vi "Generate_WayPoints_Hopping WITH VariableV2Patterning.vi"(11 "Input Cluster":T2={"Scan Rate (um/s)"=15.0, "X Start"=15.0, "X End"=15.0, "Y Start"=15.0, "Y End"=15.0, " Z Start"=15.0, "HoppingDistance"=1.0, "Voltage1"=15.0, "Z End"=15.0, "Approach Rate Hopping (um/s)"=15.0, "Retrack Rate (um/s)"=15.0, "Voltage2"=15.0, "Approach Rate (um/s)"=15.0, "Hold Time START / s"=15.0, "Hold Time Delta / s"=15.0, "Voltage1 During Retract"=0.0, "Pause on First Approach?"=FALSE, "Voltage2 During Retract"=0.0, "Voltage1 During Hold Time"=0.0, "Voltage2 During Hold Time"=0.0, "Update position loop wait time (us)"=0}) -> (1 "output cluster":T1)   [LabVIEW 2023]
uses:
  TypeDefs/WayPointCluster.ctl
  User_Vi/Settings.vi
panel:
  in  "WayPointCluster":T1
  out "Y  P":dbl
  out "X  P":dbl
  out "HoppingDistanceX":dbl
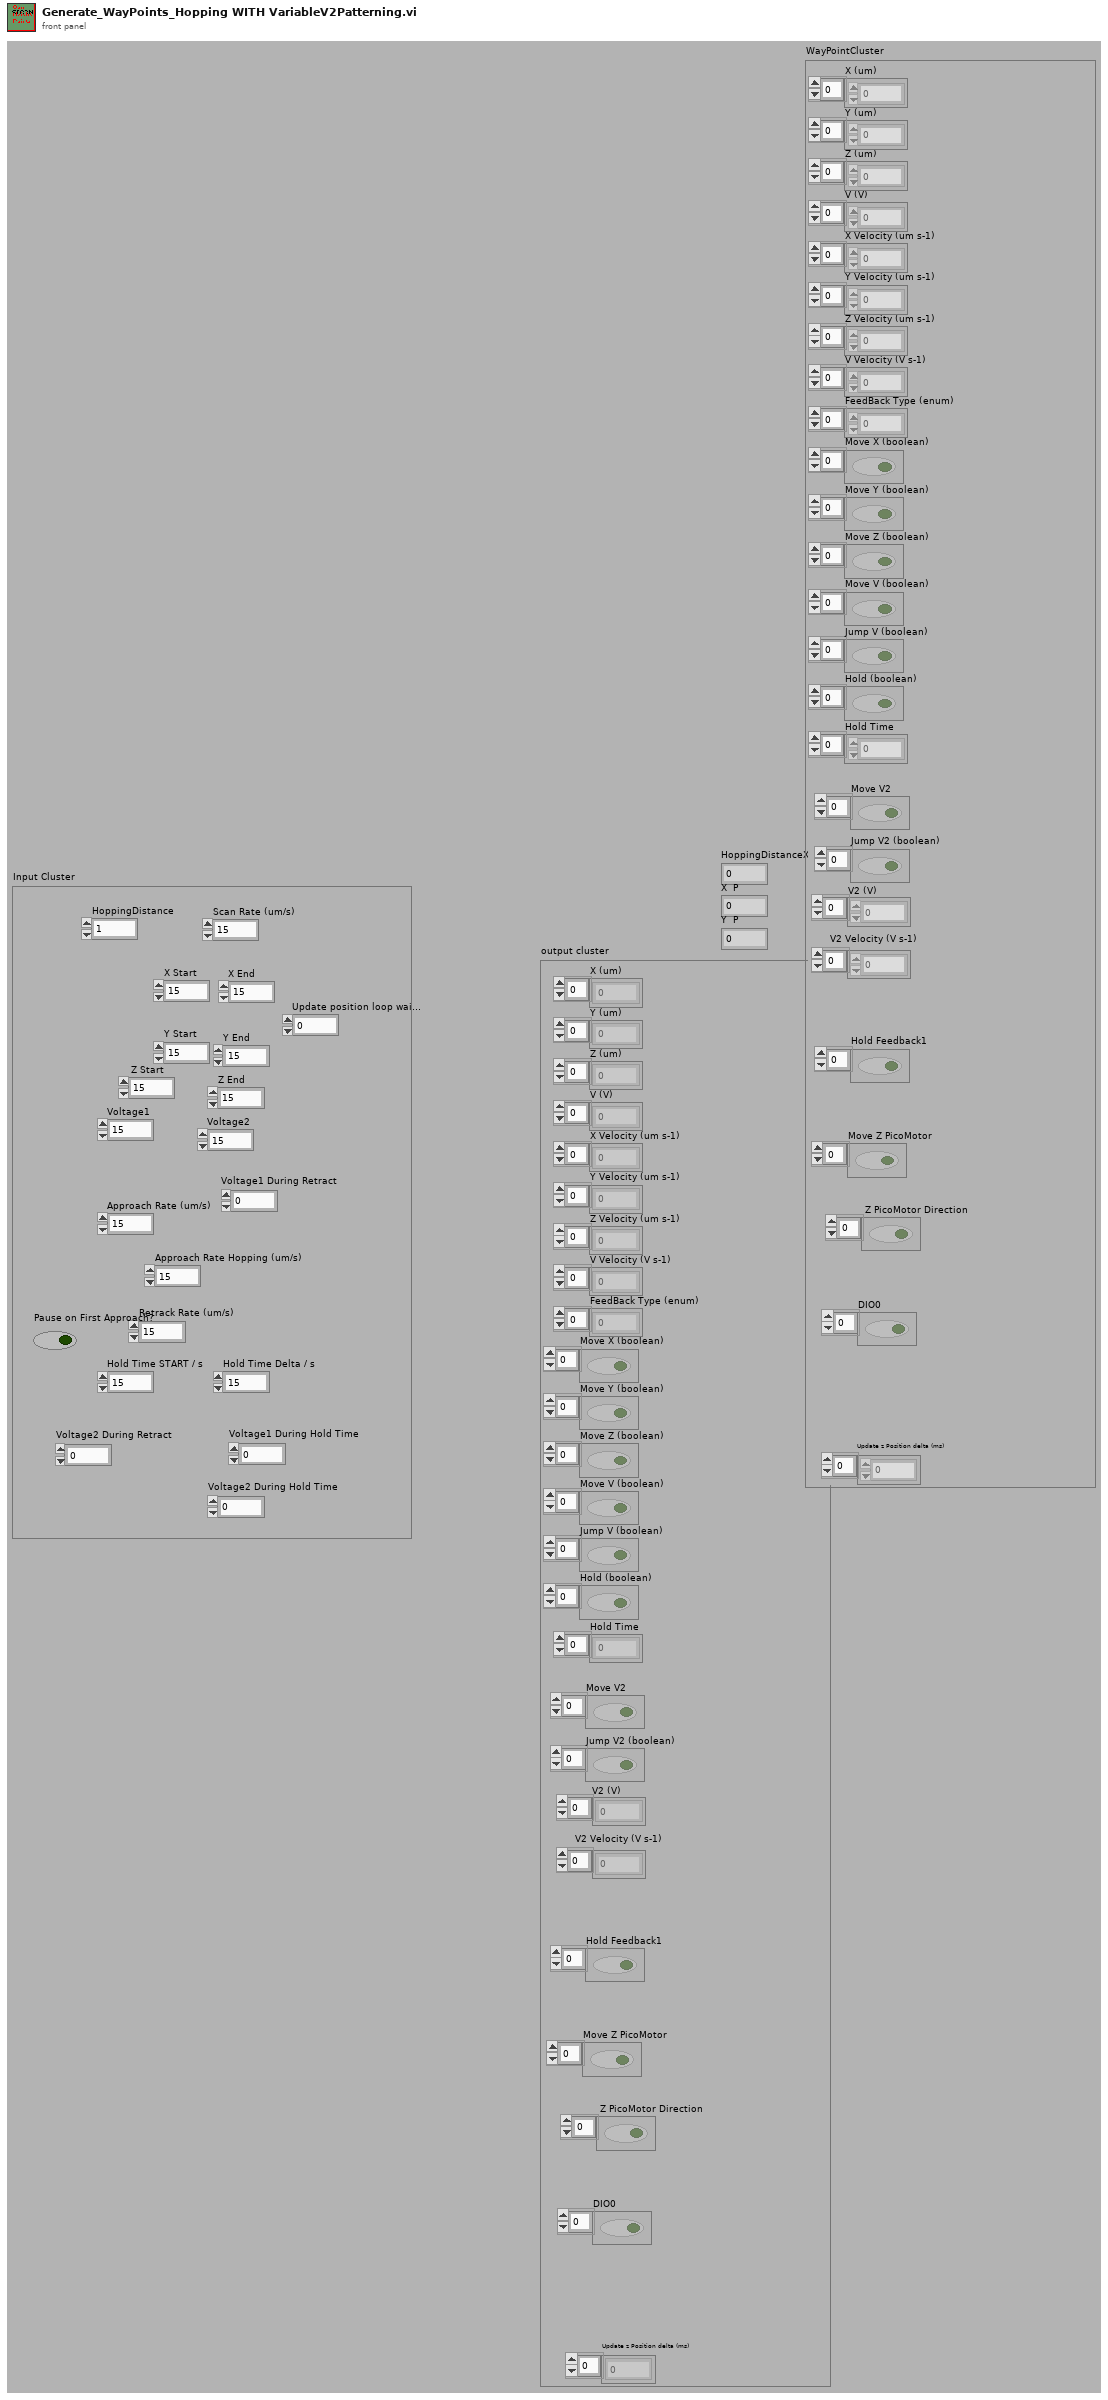
[diagram p1: front panel]
types:
  T1 = typedef "WayPointCluster.ctl" = cluster{"X (um)":dbl[], "Y (um)":dbl[], "Z (um)":dbl[], "V (V)":dbl[], "X Velocity (um s-1)":dbl[], "Y Velocity (um s-1)":dbl[], "Z Velocity (um s-1)":dbl[], "V Velocity (V s-1)":dbl[], "FeedBack Type (enum)":u16[], "Move X (boolean)":bool[], "Move Y (boolean)":bool[], "Move Z (boolean)":bool[], "Move V (boolean)":bool[], "Jump V (boolean)":bool[], "Hold (boolean)":bool[], "Hold Time":u32[], "V2 (V)":dbl[], "Move V2":bool[], "V2 Velocity (V s-1)":dbl[], "Jump V2 (boolean)":bool[], "Update z Position delta (ms)":i16[], "Hold Feedback1":bool[], "Move Z PicoMotor":bool[], " Z PicoMotor Direction":bool[], "DIO0":bool[]}
  T2 = cluster{"Scan Rate (um/s)":dbl, "X Start":dbl, "X End":dbl, "Y Start":dbl, "Y End":dbl, " Z Start":dbl, "HoppingDistance":dbl, "Voltage1":dbl, "Z End":dbl, "Approach Rate Hopping (um/s)":dbl, "Retrack Rate (um/s)":dbl, "Voltage2":dbl, "Approach Rate (um/s)":dbl, "Hold Time START / s":dbl, "Hold Time Delta / s":dbl, "Voltage1 During Retract":dbl, "Pause on First Approach?":bool, "Voltage2 During Retract":dbl, "Voltage1 During Hold Time":dbl, "Voltage2 During Hold Time":dbl, "Update position loop wait time (us)":u32}
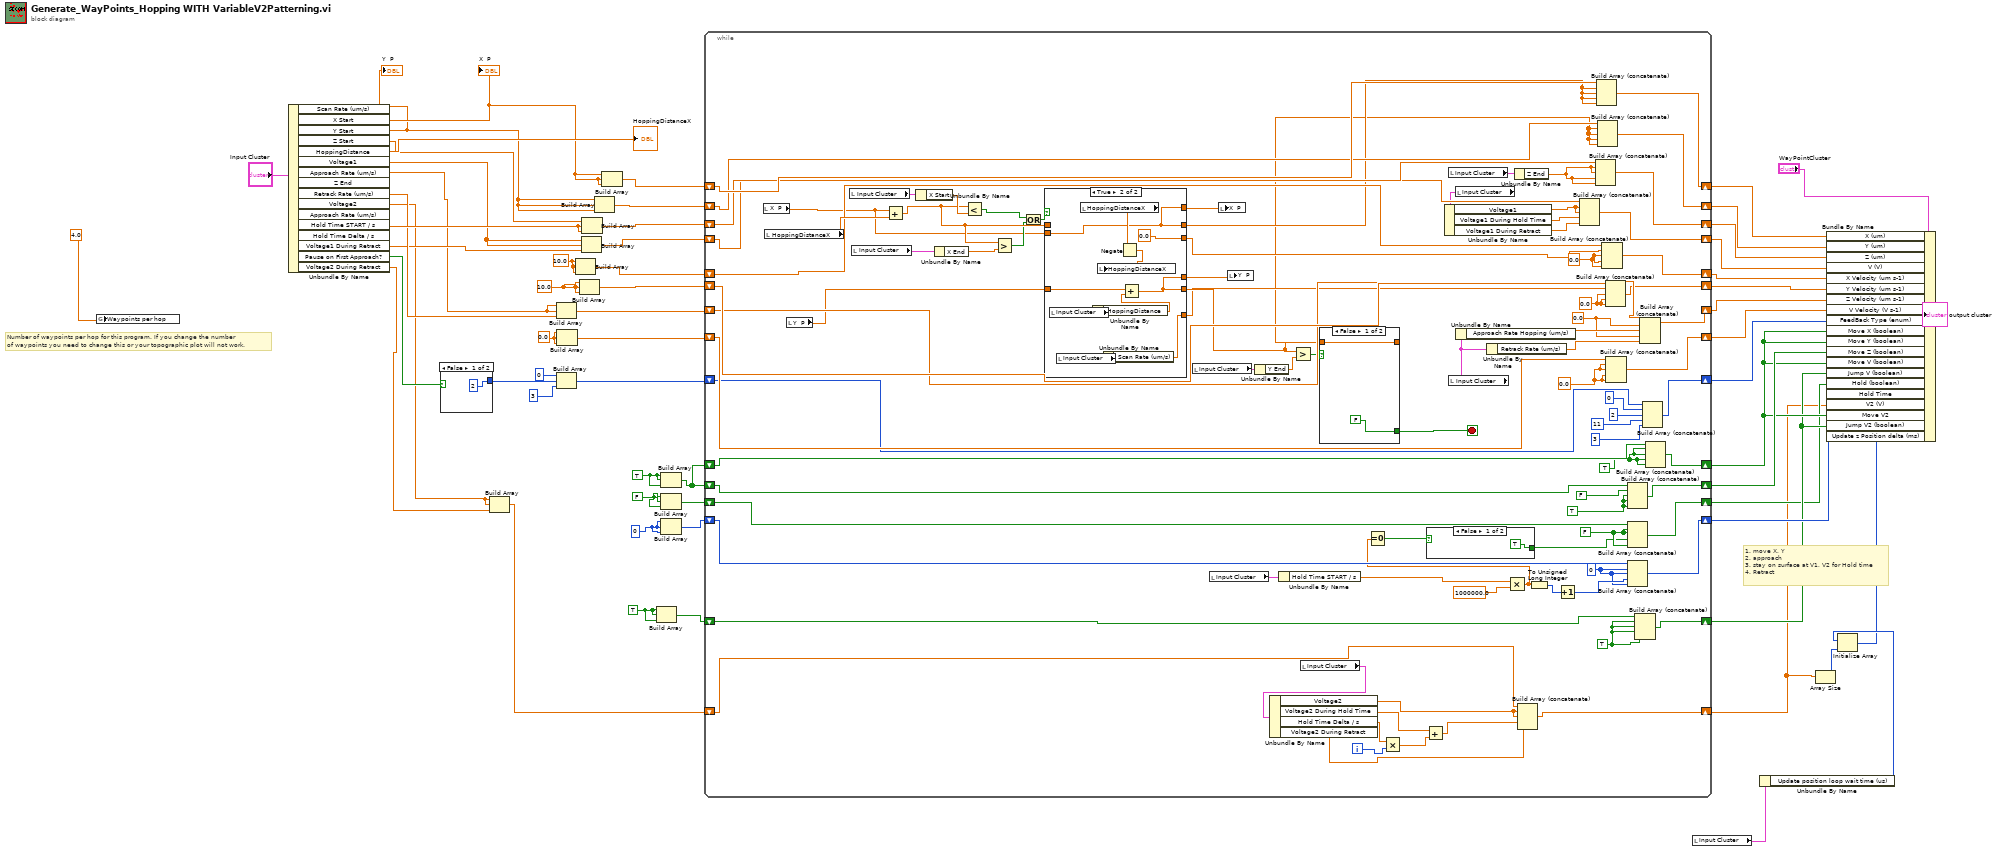
[diagram p0: block diagram]
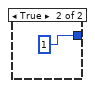
[diagram p2: hidden frame]
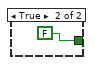
[diagram p3: hidden frame]
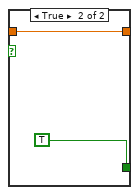
[diagram p4: hidden frame]
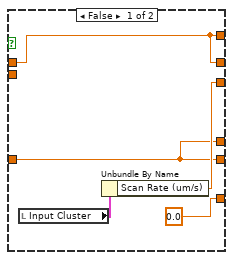
[diagram p5: hidden frame]
diagram:
  w22 = TRUE
  w23 = u32 0 ("element")
  w24 = FALSE
  w25 = TRUE
  w18 = 10.0 ("element")
  w19 = 10.0 ("element")
  w21 = 0.0 ("element")
  # "1. move X, Y\n2. approach\n3. stay on surface at V1, V2 for Hold time \n4. Retract"
  # "Number of waypoints per hop for this program. If you change the number\nof waypoints you need to change this or your topographic plot will not work."
  n1 = global write "Settings.vi" "Waypoints per hop"(4.0) -> ()
  n2 = Unbundle By Name("Input Cluster") -> ("X Start"=w39:dbl, "Y Start"=w38:dbl, "Z Start"=w40:dbl, "HoppingDistance"=→"HoppingDistanceX":dbl, "Voltage1"=w36:dbl, "Approach Rate (um/s)"=w20:dbl, "Z End"=w37:dbl, "Retrack Rate (um/s)"=w35:dbl, "Voltage2"=w12:dbl, "Voltage1 During Retract"=w27:dbl, "Pause on First Approach?"=w15:bool, "Voltage2 During Retract"=w11:dbl)  [unwired: 4 out]
  "X  P" <- w39
  "Y  P" <- w38
  n3 = case shown="False" w15 {
    tunnel: [u16 2 ("element") u16 1 ("element")] -> w14
    frame False {
    }
    frame True {
    }
  }
  n4 = Build Array(w12, w12, w11) -> (w8:dbl[])
  n5 = Build Array(w20, w20, w35) -> (w47:dbl[])
  n6 = Build Array(u16 0 ("element"), w14, u16 3 ("element")) -> (w43:u16[])
  n7 = Build Array(w21, w21, w21) -> (w45:dbl[])
  n8 = Build Array(w18, w18, w18) -> (w50:dbl[])
  n9 = Build Array(w19, w19, w19) -> (w49:dbl[])
  n10 = Build Array(w36, w36, w27) -> (w52:dbl[])
  n11 = Build Array(w40, w37, w37) -> (w54:dbl[])
  n12 = Build Array(w38, w38, w38) -> (w56:dbl[])
  n13 = Build Array(w39, w39, w39) -> (w58:dbl[])
  n14 = Build Array(w22, w22, w22) -> (w29:bool[])
  n15 = Build Array(w25, w25, w25) -> (w28:bool[])
  n16 = Build Array(w24, w24, w24) -> (w32:bool[])
  n17 = Build Array(w23, w23, w23) -> (w31:u32[])
  n18 = while {
    shift-right: [w148] -> w57
    shift-left: w58 -> [w149]
    shift-right: [w140] -> w55
    shift-left: w56 -> [w130]
    shift-right: [w139] -> w53
    shift-left: w54 -> [w147]
    shift-right: [w138] -> w51
    shift-left: w52 -> [w146]
    shift-right: [w137] -> w33
    shift-left: w50 -> [w145]
    shift-right: [w136] -> w48
    shift-left: w49 -> [w144]
    shift-right: [w135] -> w46
    shift-left: w47 -> [w143]
    shift-right: [w134] -> w44
    shift-left: w45 -> [w142]
    shift-right: [w133] -> w42
    shift-left: w43 -> [w141]
    shift-right: [w104] -> w13
    shift-left: w28 -> [w103]
    shift-right: [w105] -> w6
    shift-left: w32 -> [w109]
    shift-right: [w106] -> w30
    shift-left: w31 -> [w108]
    shift-right: [w101] -> w9
    shift-left: w29 -> [w102]
    shift-right: [w99] -> w10
    shift-left: w28 -> [w100]
    shift-right: [w84] -> w5
    shift-left: w8 -> [w85]
    i -> [w66]
    stop <- w120 stop-if-true
    w73 = TRUE
    w71 = TRUE
    w92 = u32 0 ("element")
    w94 = FALSE
    w69 = TRUE
    w77 = 0.0 ("element")
    w78 = 0.0 ("element")
    w75 = 0.0 ("element")
    w76 = 0.0 ("element")
    n19 = local read "X  P"() -> (w118:dbl)
    n20 = local read "HoppingDistanceX"() -> (w150:dbl)
    n21 = local read "Y  P"() -> (w117:dbl)
    n22 = local read "Input Cluster"() -> (w152:T2)
    n23 = local read "Input Cluster"() -> (w151:T2)
    n24 = Add(x=w118, y=w150) -> (x+y=w126:dbl)
    n25 = Unbundle By Name(w152) -> ("X Start"=w129:dbl)
    n26 = Unbundle By Name(w151) -> ("X End"=w127:dbl)
    n27 = Less?(x=w126, y=w129) -> (x < y?=w128:bool)
    n28 = Greater?(x=w126, y=w127) -> (0:w125:bool)
    n29 = Or(x=w128, y=w125) -> (x .or. y?=w124:bool)
    n30 = case shown="True" w124 {
      tunnel: w126 -> [w159 _]
      tunnel: [w159 w165] -> w82
      tunnel: w118 -> [_ w165]
      tunnel: w117 -> [w160 w166]
      tunnel: [w160 w164] -> w116
      tunnel: [w162 0.0] -> w111
      tunnel: [0.0 w167] -> w110
      tunnel: [w160 w164] -> w115
      tunnel: [w159 w165] -> w114
      frame False {
        n31 = local read "Input Cluster"() -> (w163:T2)
        n32 = Unbundle By Name(w163) -> ("Scan Rate (um/s)"=w162:dbl)
      }
      frame True {
        n33 = local read "Input Cluster"() -> (w171:T2)
        n34 = local read "Input Cluster"() -> (w169:T2)
        n35 = local read "HoppingDistanceX"() -> (w173:dbl)
        n36 = Unbundle By Name(w171) -> ("HoppingDistance"=w170:dbl)
        n37 = Unbundle By Name(w169) -> ("Scan Rate (um/s)"=w167:dbl)
        n38 = Negate(x=w173) -> (-x=w172:dbl)
        n39 = local write "HoppingDistanceX"(w172) -> ()
        n40 = Add(x=w166, y=w170) -> (x+y=w164:dbl)
      }
    }
    n41 = local read "Input Cluster"() -> (w123:T2)
    n42 = local read "Input Cluster"() -> (w107:T2)
    n43 = local write "X  P"(w114) -> ()
    n44 = local write "Y  P"(w115) -> ()
    n45 = Unbundle By Name(w123) -> ("Y End"=w122:dbl)
    n46 = Unbundle By Name(w107) -> ("Hold Time START / s"=w67:dbl)
    n47 = Greater?(x=w116, y=w122) -> (0:w121:bool)
    n48 = local read "Input Cluster"() -> (w86:T2)
    n49 = Unbundle By Name(w86) -> ("Voltage2"=w83:dbl, "Voltage2 During Hold Time"=w63:dbl, "Hold Time Delta / s"=w65:dbl, "Voltage2 During Retract"=w68:dbl)
    n50 = case shown="False" w121 {
      tunnel: w116 -> [w156 w158]
      tunnel: [w156 w158] -> w81
      tunnel: [FALSE TRUE] -> w120
      frame False {
      }
      frame True {
      }
    }
    n51 = Multiply(x=w65, y=w66) -> (x*y=w64:dbl)
    n52 = Add(x=w63, y=w64) -> (x+y=w62:dbl)
    n53 = local read "Input Cluster"() -> (w132:T2)
    n54 = local read "Input Cluster"() -> (w119:T2)
    n55 = local read "Input Cluster"() -> (w131:T2)
    n56 = Unbundle By Name(w131) -> ("Voltage1"=w88:dbl, "Voltage1 During Hold Time"=w87:dbl, "Voltage1 During Retract"=w79:dbl)
    n57 = Unbundle By Name(w119) -> ("Approach Rate Hopping (um/s)"=w112:dbl)
    n58 = Unbundle By Name(w119) -> ("Retrack Rate (um/s)"=w96:dbl)
    n59 = Multiply(x=w67, y=1000000.0) -> (x*y=w89:dbl)
    n60 = Equal To 0?(x=w89) -> (x = 0?=w90:bool)
    n61 = case shown="False" w90 {
      tunnel: [TRUE FALSE] -> w91
      frame False {
      }
      frame True {
      }
    }
    n62 = Unbundle By Name(w132) -> ("Z End"=w80:dbl)
    n63 = Build Array (concatenate)(w85, w83, w83, w62, w68) -> (w84:dbl[])
    n64 = To Unsigned Long Integer(number=w89) -> (unsigned 32bit integer=w97:u32)
    n65 = Increment(x=w97) -> (x+1=w93:u32)
    n66 = Build Array (concatenate)(w146, w88, w88, w87, w79) -> (w138:dbl[])
    n67 = Build Array (concatenate)(w147, w80, w80, w80, w80) -> (w139:dbl[])
    n68 = Build Array (concatenate)(w149, w82, w82, w82, w82) -> (w148:dbl[])
    n69 = Build Array (concatenate)(w130, w81, w81, w81, w81) -> (w140:dbl[])
    n70 = Build Array (concatenate)(w145, w111, w78, w78, w78) -> (w137:dbl[])
    n71 = Build Array (concatenate)(w144, w110, w77, w77, w77) -> (w136:dbl[])
    n72 = Build Array (concatenate)(w142, w75, w75, w75, w75) -> (w134:dbl[])
    n73 = Build Array (concatenate)(w103, FALSE, w69, w69, w69) -> (w104:bool[])
    n74 = Build Array (concatenate)(w109, w94, w94, w91, w94) -> (w105:bool[])
    n75 = Build Array (concatenate)(w108, w92, w92, w93, w92) -> (w106:u32[])
    n76 = Build Array (concatenate)(w102, w71, w71, w71, w71) -> (w101:bool[])
    n77 = Build Array (concatenate)(w143, w76, w112, w76, w96) -> (w135:dbl[])
    n78 = Build Array (concatenate)(w141, u16 0 ("element"), u16 2 ("element"), u16 11 ("element"), u16 3 ("element")) -> (w133:u16[])
    n79 = Build Array (concatenate)(w100, w73, w73, w73, w73) -> (w99:bool[])
  }
  n80 = local read "Input Cluster"() -> (w3:T2)
  n81 = Unbundle By Name(w3) -> ("Update position loop wait time (us)"=w2:u32)
  n82 = Array Size(array=w5) -> (size(s)=w4:i32)
  n83 = Initialize Array(w2, w4) -> (w1:u32[])
  n84 = Bundle By Name(cluster="WayPointCluster", "X (um)"=w57, "Y (um)"=w55, "Z (um)"=w53, "V (V)"=w51, "X Velocity (um s-1)"=w33, "Y Velocity (um s-1)"=w48, "Z Velocity (um s-1)"=w46, "V Velocity (V s-1)"=w44, "FeedBack Type (enum)"=w42, "Move X (boolean)"=w10, "Move Y (boolean)"=w10, "Move Z (boolean)"=w13, "Move V (boolean)"=w10, "Jump V (boolean)"=w9, "Hold (boolean)"=w6, "Hold Time"=w30, "V2 (V)"=w5, "Move V2"=w10, "Jump V2 (boolean)"=w9, "Update z Position delta (ms)"=w1) -> (→"output cluster":T1)
